vi "Initialize From Settings.vi"(8 "error in (no error)":errorcluster, 10 "settings":cluster{"key":string, "value":string}[](array[cluster]), 11 "Core Threads Configuration in":refnum<class "Thread Configuration.lvclass">) -> (0 "error out":errorcluster, 3 "Core Threads Configuration out":refnum<class "Thread Configuration.lvclass">)   [LabVIEW 2017, in "DSF Core.lvlib" / "Thread Configuration.lvclass"]
uses:
  Thread Configuration.lvclass
  Thread Configuration.lvclass/Thread Configuration.ctl
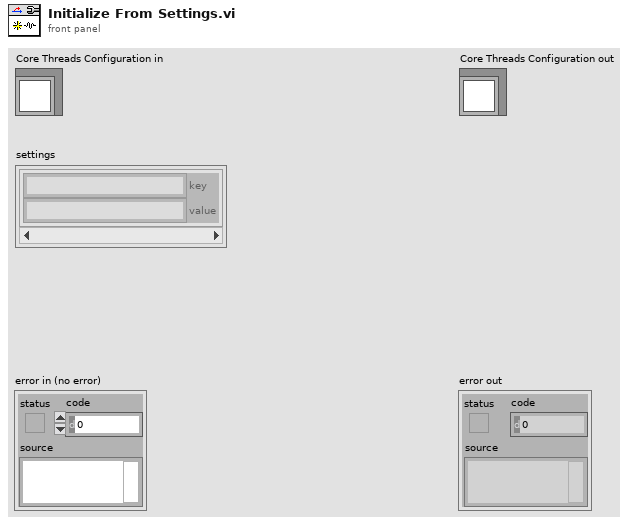
[diagram p1: front panel]
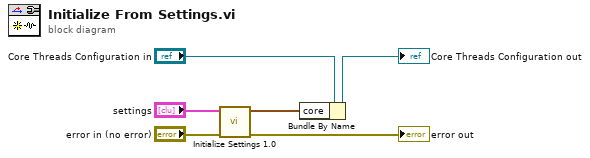
[diagram p0: block diagram]
diagram:
  n1 = call "Initialize Settings 1.0.vi"("error in (no error)"="error in (no error)", "settings 1.0"="settings") -> ("error out"=→"error out":errorcluster, "configuration 1.0"=w1:cluster{"processor":i32, "priority offset":i16})  [unwired: 8 in]
  n2 = Bundle By Name(cluster="Core Threads Configuration in", "core"=w1) -> (→"Core Threads Configuration out":refnum<class "Thread Configuration.lvclass">)
